vi "Pulse - Init DAQ Settings.vi"(8 "error in (no error)":errorcluster, 10 "Trigger Settings":T1, 11 "3300 in":refnum<class "3300.lvclass">) -> (0 "error out":errorcluster, 3 "3300 out":refnum<class "3300.lvclass">)   [LabVIEW 2019, in "3300.lvlib" / "3300.lvclass"]
uses:
  Library/3300.lvclass
  builds/Instruments/Electronic Load.lvlibp/Custom Controls/Trigger Settings.ctl
  builds/Instruments/Electronic Load.lvlibp/Custom Controls/E-Load Mode.ctl
  Library/3300.lvclass/3300.ctl
  Accessors/Read Local Resource.vi
  Accessors/Write Local Resource.vi
  <instrlib>/Agilent N330X Series/Agilent N330X Series.lvlib
  builds/Instruments/Electronic Load.lvlibp/Library/Electronic Load.lvclass
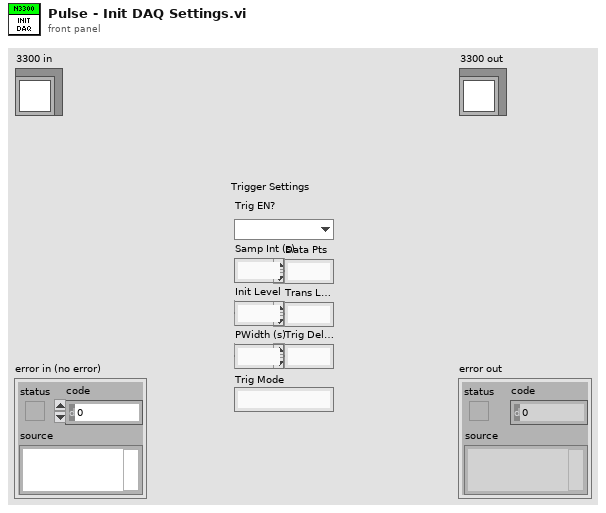
[diagram p1: front panel]
types:
  T1 = typedef "Electronic Load.lvlibp/Electronic Load.lvclass/Trigger Settings.ctl" = cluster{"Mode":T2, "Initial":dbl, "Transient":dbl, "Interval":dbl, "Width":dbl, "Delay":dbl, "Data Pts":i32, "Slew Rate":dbl}
  T2 = typedef "Electronic Load.lvlibp/Electronic Load.lvclass/E-Load Mode.ctl" = enum16{"Current", "Resistance", "Voltage"}
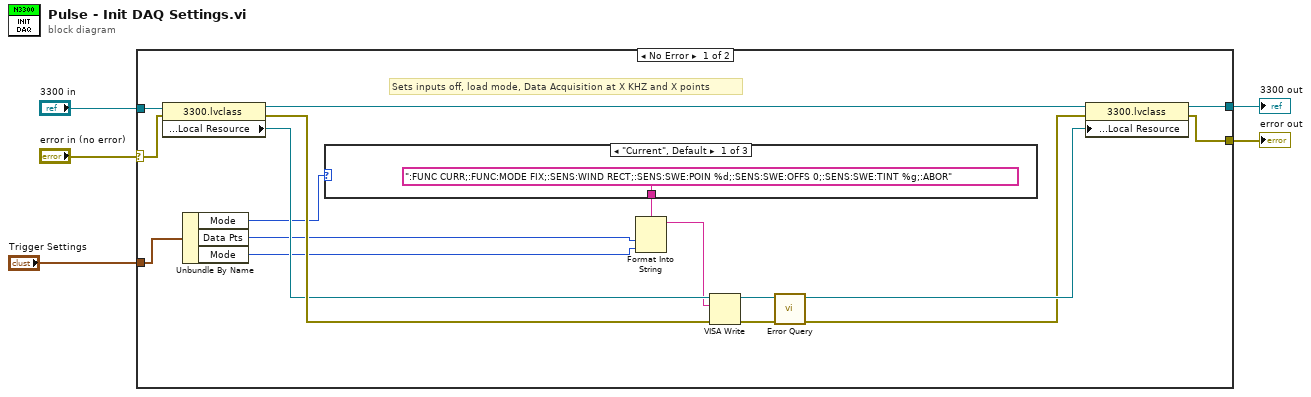
[diagram p0: block diagram]
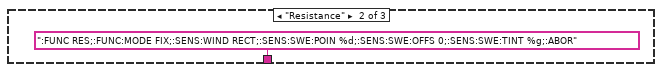
[diagram p2: hidden frame]
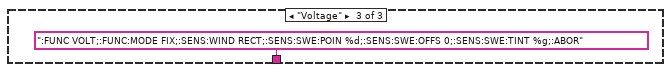
[diagram p3: hidden frame]
diagram:
  n1 = case shown="No Error" "error in (no error)" {
    selector: "error in (no error)" -> [w21 w27]
    tunnel: [w15 w27] -> w4
    tunnel: [w19 w26] -> w2
    tunnel: "3300 in" -> [w22 w26]
    tunnel: "Trigger Settings" -> [w13 _]
    frame No Error {
      # "Sets inputs off, load mode, Data Acquisition at X KHZ and X points"
      n2 = property class="3300.lvclass"(reference=w22, error in=w21) -> (reference out=w18:refnum<class "3300.lvclass">, error out=w20:errorcluster, "Private:Accessors:Local Resource"=w14:refnum<visa-resource-name>)
      n3 = Unbundle By Name(w13) -> ("Mode"=w6:T2, "Data Pts"=w11:i32, "Mode"=w10:T2)
      n4 = case shown="\"Current\", Default" w6 {
        tunnel: [":FUNC CURR;:FUNC:MODE FIX;:SENS:WIND RECT;:SENS:SWE:POIN %d;:SENS:SWE:OFFS 0;:SENS:SWE:TINT %g;:ABOR" ("string (\"\")") ":FUNC RES;:FUNC:MODE FIX;:SENS:WIND RECT;:SENS:SWE:POIN %d;:SENS:SWE:OFFS 0;:SENS:SWE:TINT %g;:ABOR" ("string (\"\")") ":FUNC VOLT;:FUNC:MODE FIX;:SENS:WIND RECT;:SENS:SWE:POIN %d;:SENS:SWE:OFFS 0;:SENS:SWE:TINT %g;:ABOR" ("string (\"\")")] -> w12
        frame "Current", Default {
        }
        frame "Resistance" {
        }
        frame "Voltage" {
        }
      }
      n5 = Format Into String(format string=w12, w11, w10) -> (resulting string=w7:string)  [unwired: 2 in, 1 out]
      n6 = VISA Write(VISA resource name=w14, write buffer=w7, error in (no error)=w20) -> (VISA resource name out=w9:refnum<visa-resource-name>, error out=w8:errorcluster)  [unwired: 1 out]
      n7 = call <instrlib>:"Error Query.vi"("error in (no error)"=w8, "VISA resource name"=w9) -> ("error out"=w16:errorcluster, "VISA resource name out"=w17:refnum<visa-resource-name>)  [unwired: 6 in, 2 out]
      n8 = property class="3300.lvclass"(reference=w18, error in=w16, "Private:Accessors:Local Resource"=w17) -> (reference out=w19:refnum<class "3300.lvclass">, error out=w15:errorcluster)
    }
    frame Error {
    }
  }
  "error out" <- w4
  "3300 out" <- w2
